vi "__Strip Path Extension - String__ogtk.vi"(0 "path":string) -> (1 "root":string, 2 "extension":string)   [LabVIEW 2019, in "LabVIEW-ClassProviderShell.lvlib"]
uses:
  LabVIEW-ClassProviderShell.lvlib
panel:
  # "Strip Path Extension.vi\n\nSplits a relative or absolute path\ninto its root and extension.  Path can be a string or a path.\n\nPlease visit http://www.OpenG.org to learn about the\nOpen Source LabVIEW software movement.\n\nNOTICE -- YOU MUST LEAVE THIS NOTICE IN PLACE.  PER THE TERMS OF THE LICENSE BELOW, YOU MAY SUBLICENSE THIS SOFTWARE \nIN ANY WAY THAT DOES NOT CONFLICT WITH THIS LICENSE.\n\n### BSD License (http://www.opensource.org/licenses/bsd-license.php) Begin ###\n \nCopyright (c) 2002, Jim Kring <jim@jimkring.com>\n\nAll rights reserved.\n\nRedistribution and use in source and binary forms, with or without modification, are permitted provided that the following conditions are met:\n\n    * Redistributions of source code must retain the above copyright notice, this list of conditions and the following disclaimer.\n    * Redistributions in binary form must reproduce the above copyright notice, this list of conditions and the following disclaimer in the \n       documentation and/or other materials provided with the distribution.\n    * Neither the name of SciWare, James Kring, Inc., nor the names of its contributors may be used to endorse or promote products derived \n       from this software without specific prior written permission.\n\nTHIS SOFTWARE IS PROVIDED BY THE COPYRIGHT HOLDERS AND CONTRIBUTORS \"AS IS\" AND ANY EXPRESS OR IMPLIED WARRANTIES, \nINCLUDING, BUT NOT LIMITED TO, THE IMPLIED WARRANTIES OF MERCHANTABILITY AND FITNESS FOR A PARTICULAR PURPOSE ARE \nDISCLAIMED. IN NO EVENT SHALL THE COPYRIGHT OWNER OR CONTRIBUTORS BE LIABLE FOR ANY DIRECT, INDIRECT, INCIDENTAL,\n SPECIAL, EXEMPLARY, OR CONSEQUENTIAL DAMAGES (INCLUDING, BUT NOT LIMITED TO, PROCUREMENT OF SUBSTITUTE GOODS OR \nSERVICES; LOSS OF USE, DATA, OR PROFITS; OR BUSINESS INTERRUPTION) HOWEVER CAUSED AND ON ANY THEORY OF LIABILITY, \nWHETHER IN CONTRACT, STRICT LIABILITY, OR TORT (INCLUDING NEGLIGENCE OR OTHERWISE) ARISING IN ANY WAY OUT OF THE USE \nOF THIS SOFTWARE, EVEN IF ADVISED OF THE POSSIBILITY OF SUCH DAMAGE.\n\n### BSD License End ###"
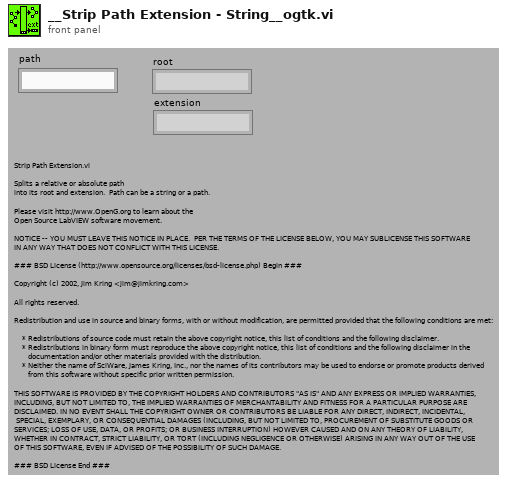
[diagram p1: front panel]
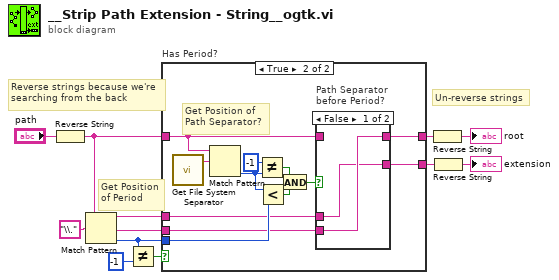
[diagram p0: block diagram]
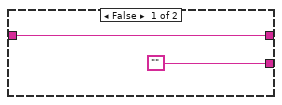
[diagram p2: hidden frame]
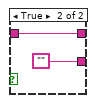
[diagram p3: hidden frame]
diagram:
  # "Get Position\nof Period"
  # "Un-reverse strings"
  # "Reverse strings because we're\nsearching from the back"
  n1 = Reverse String(1:"path") -> (0:w1:string)
  n2 = Match Pattern(string=w1, regular expression="\\.") -> (before substring=w7:string, after substring=w6:string, offset past match=w8:i32)  [unwired: 1 in, 1 out]
  n3 = Not Equal?(x=w8, y=-1) -> (x != y?=w10:bool)
  n4 = case "Has Period?" shown="True" w10 {
    tunnel: w1 -> [w14 w19]
    tunnel: ["" w17] -> w3
    tunnel: [w14 w18] -> w5
    tunnel: w8 -> [_ w23]
    tunnel: w7 -> [_ w16]
    tunnel: w6 -> [_ w15]
    frame False {
    }
    frame True {
      # "Get Position of\nPath Separator?"
      n5 = call <vilib>:"Get File System Separator.vi"() -> ("Path Separator"=w26:string)
      n6 = Match Pattern(string=w19, regular expression=w26) -> (offset past match=w24:i32)  [unwired: 1 in, 3 out]
      n7 = Not Equal?(x=-1 ("y"), y=w24) -> (x != y?=w22:bool)
      n8 = Less?(x=w24, y=w23) -> (x < y?=w21:bool)
      n9 = And(x=w22, y=w21) -> (x .and. y?=w20:bool)
      n10 = case "Path Separator\nbefore Period?" shown="False" w20 {
        tunnel: w19 -> [_ w30]
        tunnel: [w28 w30] -> w18
        tunnel: [w27 ""] -> w17
        tunnel: w16 -> [w27 _]
        tunnel: w15 -> [w28 _]
        frame False {
        }
        frame True {
        }
      }
    }
  }
  n11 = Reverse String(1:w5) -> (0:→"root":string)
  n12 = Reverse String(1:w3) -> (0:→"extension":string)
